vi "SingleAxisControlCustom.vi"() -> ()   [LabVIEW 2016, in "Aerotech VIs.lvlib"]
uses:
  Aerotech VIs.lvlib
  Motion/DisableMultiple.vi
  Motion/EnableMultiple.vi
  Motion/EnableSingle.vi
  Motion/HomeSingle.vi
  Motion/FaultAckSingle.vi
  Motion/DisableSingle.vi
  Motion/AbortSingle.vi
  Motion/MoveIncSingle.vi
  Motion/FreerunSingle.vi
  Parameters/GetAxisParameterString.vi
  Parameters/GetAxisParameterDouble.vi
panel:
  in  "axis":i32
  in  "Joystick":bool
  in  "Disconnect?":bool
  in  "taskId":i32(ring)=1 items=["TLibrary", "T01", "T02", "T03", "T04", "T05", "T06", "T07", "T08", "T09", "T10", "T11", "T12", "T13", "T14", "T15", "T16", "T17", "T18", "T19", "T20", "T21", "T22", "T23", "T24", "T25", "T26", "T27", "T28", "T29", "T30", "T31"]
  in  "Abort":bool
  out "do stop":bool
  out "Vel Units":string
  out "Pos Units":string
  in  "stop":bool
  out "Vel Fbk":dbl
  out "Pos Fbk":dbl
  out "Status":string
  in  "Jog Right":bool
  in  "Jog Left":bool
  in  "Distance":dbl=1000.0 min=0.0 max=360.0
  in  "Speed":dbl=5000.0 min=0.0 max=36.0
  in  "Jog":bool
  in  "FaultAck":bool
  in  "Home":bool
  in  "Disable":bool
  in  "Enable":bool
  out "Axis":string
  # "Don't use joystick when jog in progress"
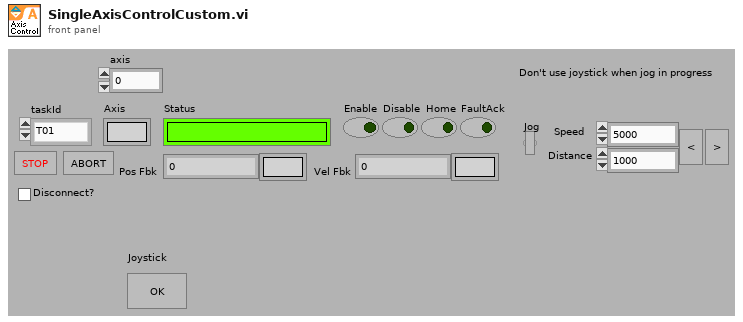
[diagram p1: front panel]
types:
  T1 = cluster{"new reference":refnum<k24>, "Event Callback":refnum<k27>, "ControllerDiagPacket":refnum<user-event>, "Event Registration Refnum":refnum<event-registration>}
  T2 = typedef "AxisDiagPacket.ctl" = cluster{"Axis Name":string, "Analog Input 0":dbl, "Analog Input 1":dbl, "Axis Fault (num)":i32, "Axis Fault (str)":string, "Axis Fault (bits)":cluster{"AmplifierFault":bool, "AmplifierTemperatureFault":bool, "CcwEndOfTravelLimitFault":bool, "CcwSoftwareLimitFault":bool, "CommunicationLostFault":bool, "CwEndOfTravelLimitFault":bool, "CwSoftwareLimitFault":bool, "EmergencyStopFault":bool, "EncoderFault":bool, "ExternalFault":bool, "FeedbackScalingFault":bool, "GantryMisalignFault ":bool, "HallSensorFault":bool, "InPositionTimeoutFault":bool, "MarkerSearchFault":bool, "MaxVelocityCommandFault":bool, "MotorTemperatureFault":bool, "None":bool, "OverCurrentFault":bool, "PositionErrorFault":bool, "PositionFeedbackFault":bool, "ProbeInputFault":bool, "SafeZoneFault":bool, "VelocityErrorFault":bool, "VelocityFeedbackFault":bool, "VoltageClampFault":bool, "PowerSupplyFault":bool}, "Axis Status (num)":i32, "Axis Status (str)":string, "Axis Status (bits)":cluster{"BacklashActive":bool, "CalibrationEnabled1D":bool, "CalibrationEnabled2D":bool, "CommandValid":bool, "DriveAbortPending":bool, "DrivePending":bool, "Enabling":bool, "GainMappingEnabled":bool, "GantryAligned":bool, "GantryRealigning":bool, "Homed":bool, "Homing":bool, "IFOVEnabled":bool, "Jogging":bool, "JogGenerating":bool, "JoystickControl":bool, "MasterSlaveControl":bool, "MotionBlocked":bool, "MotionClamped":bool, "MoveDone":bool, "None":bool, "NotVirtual":bool, "Profiling":bool, "Stability0":bool, "Stability1":bool, "TrajectoryFiltering":bool, "WaitDone":bool}, "Current Command":sgl, "Current Error":sgl, "Current Feedback":sgl, "Digital Inputs":i32, "Digital Outputs":i32, "Drive Status":i32, "Drive Status (str)":string, "Drive Status (bits)":cluster{"AccelerationPhase":bool, "AutofocusActive":bool, "BrakeOutput":bool, "CcwEndOfTravelLimitInput":bool, "CosineEncoderError":bool, "CurrentClamp":bool, "CwEndOfTravelLimitInput":bool, "DecelerationPhase":bool, "DualLoopActive":bool, "EmergencyStopInput":bool, "Enabled":bool, "EncoderClipping":bool, "GalvoCalibrationEnabled":bool, "GalvoPowerCorrection":bool, "HallAInput":bool, "HallBInput":bool, "HallCInput":bool, "HighResolutionMode":bool, "HomeLimitInput":bool, "InPosition":bool, "InPosition2":bool, "MarkerInput":bool, "MarkerLatch":bool, "MoveActive":bool, "NoMotorSupply":bool, "None":bool, "PowerLimiting":bool, "ProgrammingFlash":bool, "ProgrammingMXH":bool, "PSOHaltLatch":bool, "ServoControl":bool, "SineEncoderError":bool}, "Position Feedback Auxiliary":dbl, "Position Command":dbl, "Position Error":dbl, "Position Feedback":dbl, "Program Position Command":dbl, "Program Position Error":dbl, "Program Position Feedback":dbl, "Velocity Command":dbl, "Velocity Error":dbl, "Velocity Feedback":dbl}
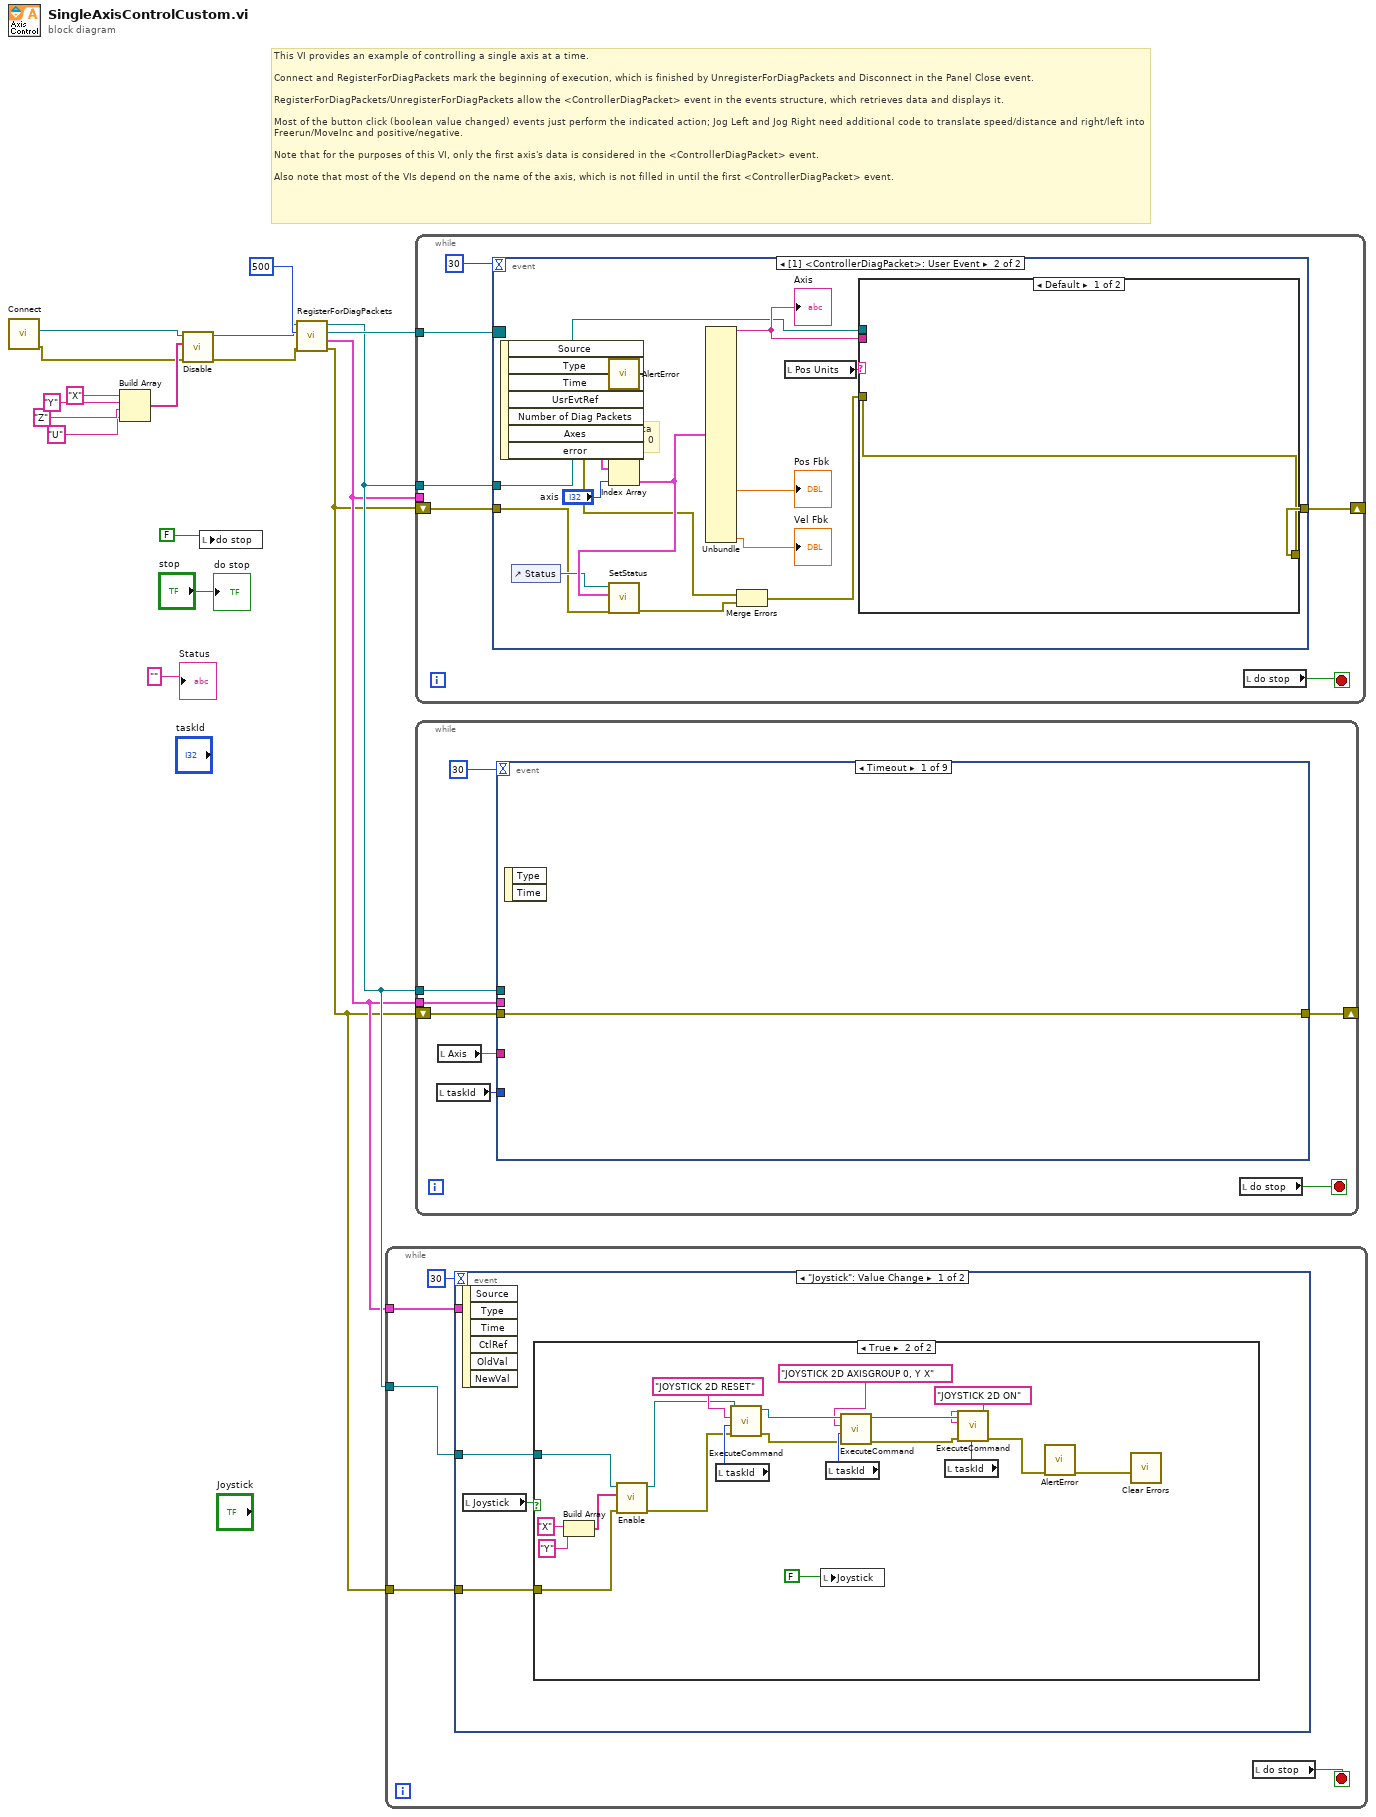
[diagram p0: block diagram]
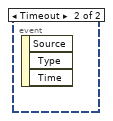
[diagram p3: hidden frame]
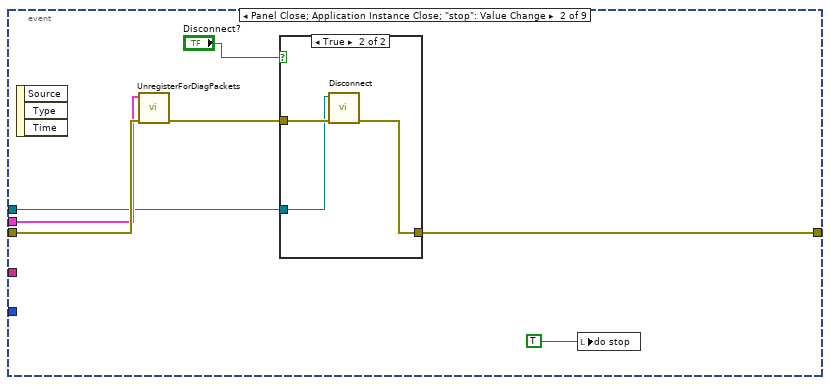
[diagram p4: hidden frame]
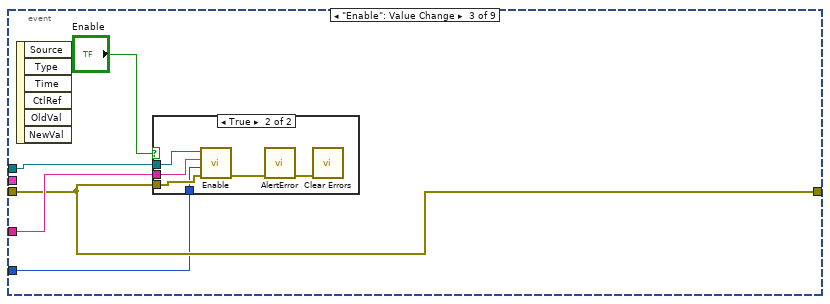
[diagram p6: hidden frame]
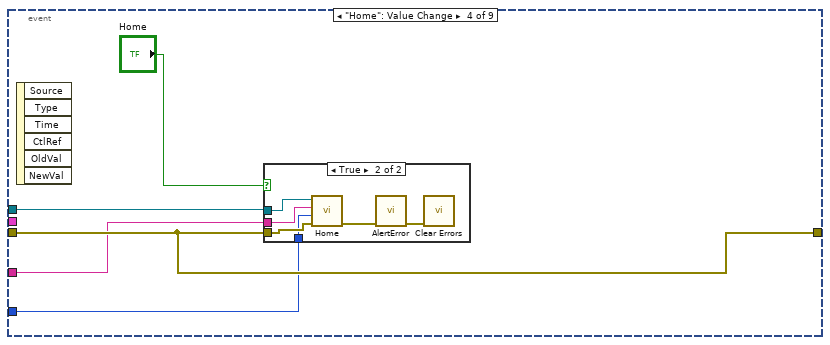
[diagram p8: hidden frame]
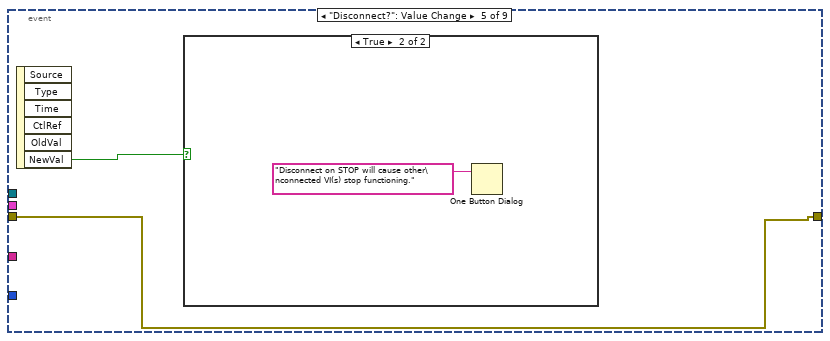
[diagram p10: hidden frame]
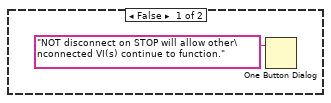
[diagram p11: hidden frame]
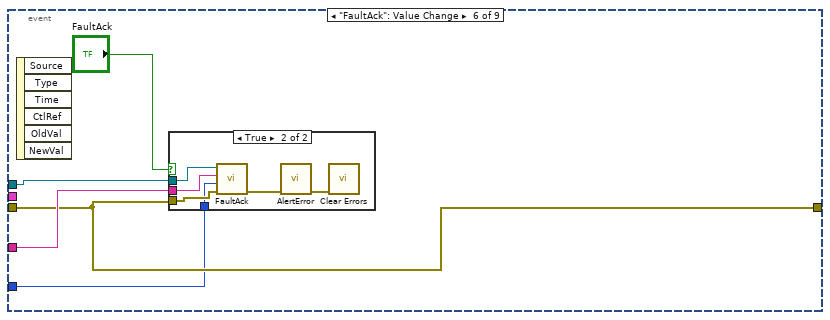
[diagram p12: hidden frame]
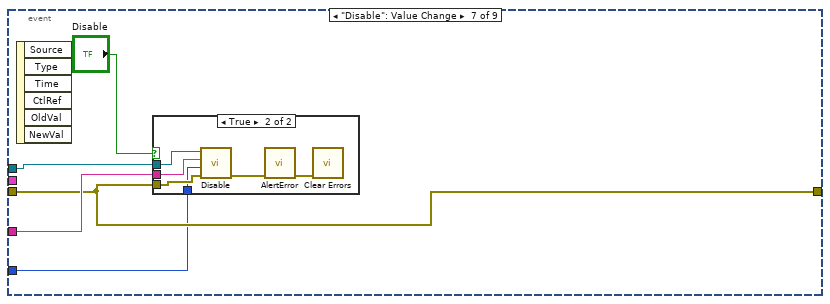
[diagram p14: hidden frame]
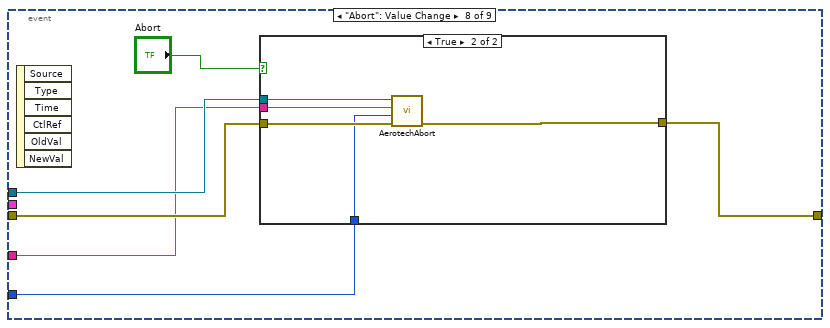
[diagram p16: hidden frame]
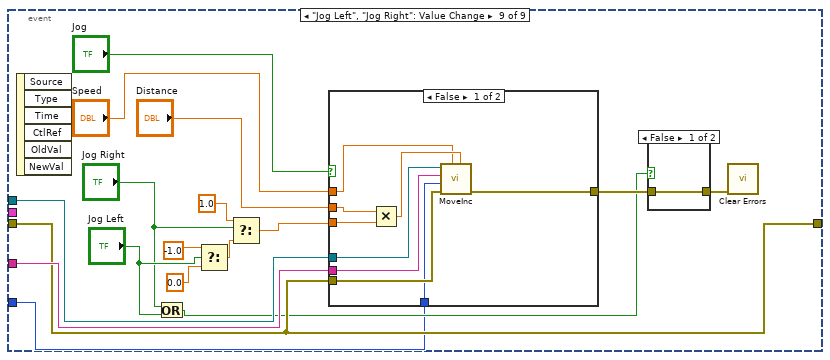
[diagram p18: hidden frame]
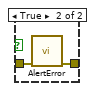
[diagram p19: hidden frame]
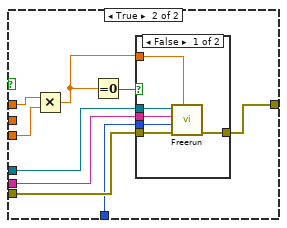
[diagram p20: hidden frame]
diagram:
  # "This VI provides an example of controlling a single axis at a time. \n\nConnect and RegisterForDiagPackets mark the beginning of execution, which is finished by UnregisterForDiagPackets and Disconnect in the Panel Close event.\n\nRegisterForDiagPackets/UnregisterForDiagPackets allow the <ControllerDiagPacket> event in the events structure, which retrieves data and displays it.\n\nMost of the button click (boolean value changed) events just perform the indicated action; Jog Left and Jog Right need additional code to translate speed/distance and right/left into Freerun/MoveInc and positive/negative.\n\nNote that for the purposes of this VI, only the first axis's data is considered in the <ControllerDiagPacket> event.\n\nAlso note that most of the VIs depend on the name of the axis, which is not filled in until the first <ControllerDiagPacket> event."
  n1 = call "Connect.vi"() -> ("error out"=w6:errorcluster, "controller"=w7:refnum<k24>)  [unwired: 10 in]
  n2 = Build Array("X", "Y", "Z", "U") -> (w8:string[])
  n3 = call-poly "Disable.vi"("error in (no error)"=w6, "axis names"=w8, "controller in"=w7) -> ("error out"=w11:errorcluster, "controller out"=w12:refnum<k24>)  [unwired: 7 in]
  n4 = local write "do stop"(FALSE ("do stop")) -> ()
  n5 = call "RegisterForDiagPackets.vi"("error in (no error)"=w11, "refresh interval (default)"=500, "Controller in"=w12) -> ("error out"=w1:errorcluster, "Event Metadata"=w2:T1, "Event Registration Refnum"=w17:refnum<event-registration>, "Controller out"=w3:refnum<k24>)  [unwired: 4 in]
  n6 = while {
    tunnel: w3 -> [w22]
    tunnel: w2 -> [w20]
    tunnel: w1 -> [w18]
    stop <- w21 stop-if-true
    n7 = event shown="[0] \"Joystick\": Value Change" {
      selector: _ -> [_ _]
      dyn-events: _ -> [_ _]
      timeout: 30 -> [_ _]
      tunnel: w22 -> [w25 _]
      tunnel: w20 -> [_ _]
      tunnel: w18 -> [w23 _]
      event "Joystick": Value Change {
        n8 = event-data() -> ()  [unwired: 1 in, 6 out]
        n9 = local read "Joystick"() -> (w24:bool)
        n10 = case shown="True" w24 {
          tunnel: w25 -> [_ w28]
          tunnel: w23 -> [_ w27]
          frame False {
          }
          frame True {
            n11 = Build Array("X", "Y") -> (w34:string[])
            n12 = call-poly "Enable.vi"("error in (no error)"=w27, "axis names"=w34, "controller in"=w28) -> ("error out"=w32:errorcluster, "controller out"=w33:refnum<k24>)  [unwired: 7 in]
            n13 = local read "taskId"() -> (w42:i32)
            n14 = call "ExecuteCommand.vi"("error in (no error)"=w32, "taskId"=w42, "Command Code"="JOYSTICK 2D RESET", "controller in"=w33) -> ("error out"=w38:errorcluster, "controller out"=w40:refnum<k24>)  [unwired: 5 in, 1 out]
            n15 = local write "Joystick"(FALSE) -> ()
            n16 = local read "taskId"() -> (w43:i32)
            n17 = call "ExecuteCommand.vi"("error in (no error)"=w38, "taskId"=w43, "Command Code"="JOYSTICK 2D AXISGROUP 0, Y X", "controller in"=w40) -> ("error out"=w39:errorcluster, "controller out"=w41:refnum<k24>)  [unwired: 5 in, 1 out]
            n18 = local read "taskId"() -> (w44:i32)
            n19 = call "ExecuteCommand.vi"("error in (no error)"=w39, "taskId"=w44, "Command Code"="JOYSTICK 2D ON", "controller in"=w41) -> ("error out"=w45:errorcluster)  [unwired: 5 in, 2 out]
            n20 = call "AlertError.vi"("error in (no error)"=w45) -> ("error out"=w29:errorcluster)  [unwired: 10 in]
            n21 = call <vilib>:"Clear Errors.vi"("error in (no error)"=w29) -> ()  [unwired: 5 in, 2 out]
          }
        }
      }
      event Timeout {
        n22 = event-data() -> ()  [unwired: 1 in, 3 out]
      }
    }
    n23 = local read "do stop"() -> (w21:bool)
  }
  n24 = while {
    tunnel: w17 -> [w46]
    tunnel: w2 -> [_]
    tunnel: w3 -> [w50]
    shift-right: [w48] -> _
    shift-left: w1 -> [w49]
    stop <- w47 stop-if-true
    n25 = event shown="[1] <ControllerDiagPacket>: User Event" {
      selector: w46 -> [_ _]
      dyn-events: _ -> [_ _]
      timeout: 30 -> [_ _]
      tunnel: w50 -> [_ w57]
      tunnel: w49 -> [w52 w56]
      tunnel: [w52 w55] -> w48
      event Timeout {
        n26 = event-data() -> ()  [unwired: 1 in, 2 out]
      }
      event User Event {
        # "Get data for axis 0"
        n27 = event-data() -> ("Axes"=w59:T2[], "error"=w58:errorcluster)  [unwired: 1 in, 5 out]
        n28 = control-ref of="Status"() -> (w61:refnum<vi>)
        n29 = call "AlertError.vi"("error in (no error)"=w58) -> ()  [unwired: 10 in, 1 out]
        n30 = Index Array(array=w59, index="axis") -> (element=w62:T2)
        n31 = call "SetStatus.vi"("error in (no error)"=w56, "AxisDiagPacket"=w62, "Status string"=w61) -> ("error out"=w63:errorcluster)  [unwired: 8 in]
        n32 = Unbundle(w62) -> ("Axis Name"=w64:string, "Position Feedback"=→"Pos Fbk":dbl, "Velocity Feedback"=→"Vel Fbk":dbl)  [unwired: 24 out]
        "Axis" <- w64
        n33 = Merge Errors(w58, w63) -> (w65:errorcluster)
        n34 = local read "Pos Units"() -> (w66:string)
        n35 = case shown="Default" w66 {
          tunnel: w64 -> [_ w80]
          tunnel: w57 -> [_ w81]
          tunnel: w65 -> [w67 w85]
          tunnel: [w67 w75] -> w55
          frame Default {
          }
          frame "" {
            w68 = 2.0 ("y")
            # "Set display units and max jog speed/distance if not yet set"
            n36 = call-poly "GetAxisParameter.vi"("error in (no error)"=w85, "Parameter Name"="UnitsName" ("parameter name"), "axis name"=w80, "controller in"=w81) -> ("error out"=w82:errorcluster, "value"=w86:string)  [unwired: 5 in, 1 out]
            "Pos Units" <- w86
            n37 = call-poly "GetAxisParameter.vi"("error in (no error)"=w82, "Parameter Name"="MaxJogSpeed" ("parameter name"), "axis name"=w80, "controller in"=w81) -> ("error out"=w83:errorcluster, "value"=w70:dbl)  [unwired: 5 in, 1 out]
            n38 = call-poly "GetAxisParameter.vi"("error in (no error)"=w83, "Parameter Name"="MaxJogDistance" ("parameter name"), "axis name"=w80, "controller in"=w81) -> ("error out"=w73:errorcluster, "value"=w69:dbl)  [unwired: 5 in, 1 out]
            n39 = Divide(x=w70, y=w68) -> (x/y=w71:dbl)
            n40 = Divide(x=w69, y=w68) -> (x/y=w72:dbl)
            n41 = control-ref of="Distance"() -> (w76:refnum<vi>)
            n42 = control-ref of="Speed"() -> (w77:refnum<vi>)
            n43 = Concatenate Strings(w86, "/s" ("string")) -> (→"Vel Units":string)
            n44 = property class="DigNum (strict)"(reference=w77, error in=w73, "Value"=w71, "Maximum"=w70) -> (error out=w74:errorcluster)  [unwired: 1 out]
            n45 = property class="DigNum (strict)"(reference=w76, error in=w74, "Value"=w72, "Maximum"=w69) -> (error out=w75:errorcluster)  [unwired: 1 out]
          }
        }
      }
    }
    n46 = local read "do stop"() -> (w47:bool)
  }
  n47 = while {
    tunnel: w3 -> [w92]
    shift-right: [w89] -> _
    shift-left: w1 -> [w96]
    tunnel: w2 -> [w91]
    stop <- w93 stop-if-true
    n48 = local read "taskId"() -> (w90:i32)
    n49 = local read "Axis"() -> (w95:string)
    n50 = event shown="[0] Timeout" {
      selector: _ -> [_ _ _ _ _ _ _ _ _]
      dyn-events: _ -> [_ _ _ _ _ _ _ _ _]
      timeout: 30 -> [_ _ _ _ _ _ _ _ _]
      tunnel: w92 -> [_ w98 w113 w120 _ w139 w149 w160 w176]
      tunnel: w96 -> [w97 w100 w110 w124 w131 w137 w147 w161 w175]
      tunnel: w95 -> [_ _ w112 w123 _ w138 w148 w158 w177]
      tunnel: w91 -> [_ w99 _ _ _ _ _ _ _]
      tunnel: w90 -> [_ _ w109 w122 _ w135 w146 w157 w169]
      tunnel: [w97 w104 w110 w124 w131 w137 w147 w159 w175] -> w89
      event Timeout {
        n51 = event-data() -> ()  [unwired: 1 in, 2 out]
      }
      event Panel Close; Application Instance Close; "stop": Value Change {
        n52 = event-data() -> ()  [unwired: 1 in, 3 out]
        n53 = call "UnregisterForDiagPackets.vi"("Event Metadata"=w99, "error in (no error)"=w100) -> ("error out"=w101:errorcluster)  [unwired: 8 in]
        n54 = case shown="True" "Disconnect?" {
          tunnel: w101 -> [w105 w108]
          tunnel: [w105 w107] -> w104
          tunnel: w98 -> [_ w106]
          frame False {
          }
          frame True {
            n55 = call "Disconnect.vi"("error in (no error)"=w108, "controller"=w106) -> ("error out"=w107:errorcluster)  [unwired: 9 in]
          }
        }
        n56 = local write "do stop"(TRUE) -> ()
      }
      event "Enable": Value Change {
        n57 = event-data() -> ()  [unwired: 1 in, 6 out]
        n58 = case shown="True" "Enable" {
          tunnel: w113 -> [_ w118]
          tunnel: w110 -> [_ w116]
          tunnel: w112 -> [_ w117]
          tunnel: w109 -> [_ w114]
          frame False {
          }
          frame True {
            n59 = call-poly "Enable.vi"("error in (no error)"=w116, "taskId"=w114, "axis name"=w117, "controller in"=w118) -> ("error out"=w115:errorcluster)  [unwired: 6 in, 1 out]
            n60 = call "AlertError.vi"("error in (no error)"=w115) -> ("error out"=w119:errorcluster)  [unwired: 10 in]
            n61 = call <vilib>:"Clear Errors.vi"("error in (no error)"=w119) -> ()  [unwired: 5 in, 2 out]
          }
        }
      }
      event "Home": Value Change {
        n62 = event-data() -> ()  [unwired: 1 in, 6 out]
        n63 = case shown="True" "Home" {
          tunnel: w120 -> [_ w130]
          tunnel: w124 -> [_ w128]
          tunnel: w123 -> [_ w129]
          tunnel: w122 -> [_ w125]
          frame False {
          }
          frame True {
            n64 = call-poly "Home.vi"("error in (no error)"=w128, "taskId"=w125, "axis name"=w129, "controller in"=w130) -> ("error out"=w127:errorcluster)  [unwired: 6 in, 1 out]
            n65 = call "AlertError.vi"("error in (no error)"=w127) -> ("error out"=w126:errorcluster)  [unwired: 10 in]
            n66 = call <vilib>:"Clear Errors.vi"("error in (no error)"=w126) -> ()  [unwired: 5 in, 2 out]
          }
        }
      }
      event "Disconnect?": Value Change {
        n67 = event-data() -> ("NewVal"=w132:bool)  [unwired: 1 in, 5 out]
        n68 = case shown="True" w132 {
          frame False {
            n69 = One Button Dialog(message="NOT disconnect on STOP will allow other\nconnected VI(s) continue to function.") -> ()  [unwired: 1 in, 1 out]
          }
          frame True {
            n70 = One Button Dialog(message="Disconnect on STOP will cause other\nconnected VI(s) stop functioning.") -> ()  [unwired: 1 in, 1 out]
          }
        }
      }
      event "FaultAck": Value Change {
        n71 = event-data() -> ()  [unwired: 1 in, 6 out]
        n72 = case shown="True" "FaultAck" {
          tunnel: w139 -> [_ w145]
          tunnel: w137 -> [_ w143]
          tunnel: w138 -> [_ w144]
          tunnel: w135 -> [_ w140]
          frame False {
          }
          frame True {
            n73 = call-poly "FaultAck.vi"("error in (no error)"=w143, "taskId"=w140, "axis name"=w144, "controller in"=w145) -> ("error out"=w142:errorcluster)  [unwired: 6 in, 1 out]
            n74 = call "AlertError.vi"("error in (no error)"=w142) -> ("error out"=w141:errorcluster)  [unwired: 10 in]
            n75 = call <vilib>:"Clear Errors.vi"("error in (no error)"=w141) -> ()  [unwired: 5 in, 2 out]
          }
        }
      }
      event "Disable": Value Change {
        n76 = event-data() -> ()  [unwired: 1 in, 6 out]
        n77 = case shown="True" "Disable" {
          tunnel: w149 -> [_ w156]
          tunnel: w147 -> [_ w154]
          tunnel: w148 -> [_ w155]
          tunnel: w146 -> [_ w151]
          frame False {
          }
          frame True {
            n78 = call-poly "Disable.vi"("error in (no error)"=w154, "taskId"=w151, "axis name"=w155, "controller in"=w156) -> ("error out"=w153:errorcluster)  [unwired: 6 in, 1 out]
            n79 = call "AlertError.vi"("error in (no error)"=w153) -> ("error out"=w152:errorcluster)  [unwired: 10 in]
            n80 = call <vilib>:"Clear Errors.vi"("error in (no error)"=w152) -> ()  [unwired: 5 in, 2 out]
          }
        }
      }
      event "Abort": Value Change {
        n81 = event-data() -> ()  [unwired: 1 in, 6 out]
        n82 = case shown="True" "Abort" {
          tunnel: w160 -> [_ w168]
          tunnel: w161 -> [w163 w167]
          tunnel: [w163 w166] -> w159
          tunnel: w158 -> [_ w165]
          tunnel: w157 -> [_ w164]
          frame False {
          }
          frame True {
            n83 = call-poly "AerotechAbort.vi"("error in (no error)"=w167, "taskId"=w164, "axis name? (all)"=w165, "controller in"=w168) -> ("error out"=w166:errorcluster)  [unwired: 6 in, 1 out]
          }
        }
      }
      event "Jog Left", "Jog Right": Value Change {
        n84 = event-data() -> ()  [unwired: 1 in, 6 out]
        n85 = Or(x="Jog Right", y="Jog Left") -> (x .or. y?=w170:bool)
        n86 = Select(t=-1.0, s="Jog Left", f=0.0) -> (s? t:f=w185:dbl)
        n87 = Select(t=1.0, s="Jog Right", f=w185) -> (s? t:f=w181:dbl)
        n88 = case shown="False" "Jog" {
          tunnel: "Speed" -> [w192 w206]
          tunnel: "Distance" -> [w197 _]
          tunnel: w181 -> [w196 w205]
          tunnel: w175 -> [w195 w204]
          tunnel: w177 -> [w191 w203]
          tunnel: w176 -> [w190 w202]
          tunnel: [w194 w201] -> w173
          tunnel: w169 -> [w189 w200]
          frame False {
            n89 = Multiply(x=w197, y=w196) -> (x*y=w193:dbl)
            n90 = call-poly "MoveInc.vi"("distance"=w193, "speed"=w192, "error in (no error)"=w195, "taskId"=w189, "axis name"=w191, "controller in"=w190) -> ("error out"=w194:errorcluster)  [unwired: 4 in, 1 out]
          }
          frame True {
            n91 = Multiply(x=w206, y=w205) -> (x*y=w198:dbl)
            n92 = Equal To 0?(x=w198) -> (x = 0?=w199:bool)
            n93 = case shown="False" w199 {
              tunnel: w204 -> [w212 w217]
              tunnel: w203 -> [w211 w214]
              tunnel: w202 -> [w210 w215]
              tunnel: [w209 w216] -> w201
              tunnel: w198 -> [w208 _]
              tunnel: w200 -> [w207 w213]
              frame False {
                n94 = call-poly "Freerun.vi"("speed"=w208, "error in (no error)"=w212, "taskId"=w207, "axis name"=w211, "controller in"=w210) -> ("error out"=w209:errorcluster)  [unwired: 5 in, 1 out]
              }
              frame True {
                n95 = call-poly "AerotechAbort.vi"("error in (no error)"=w217, "taskId"=w213, "axis name? (all)"=w214, "controller in"=w215) -> ("error out"=w216:errorcluster)  [unwired: 6 in, 1 out]
              }
            }
          }
        }
        n96 = case shown="False" w170 {
          tunnel: [w186 w188] -> w174
          tunnel: w173 -> [w186 w187]
          frame False {
          }
          frame True {
            n97 = call "AlertError.vi"("error in (no error)"=w187) -> ("error out"=w188:errorcluster)  [unwired: 10 in]
          }
        }
        n98 = call <vilib>:"Clear Errors.vi"("error in (no error)"=w174) -> ()  [unwired: 5 in, 2 out]
      }
    }
    n99 = local read "do stop"() -> (w93:bool)
  }
  "Status" <- "" ("Status")
  "do stop" <- "stop"
